vi "temp22100.vi"() -> ()   [LabVIEW 2010]
panel:
  out "Waveform Chart":dbl(graph)
  in  "Boolean":bool
  in  "stop":bool
  in  "Delay Time (s)":dbl=1.0
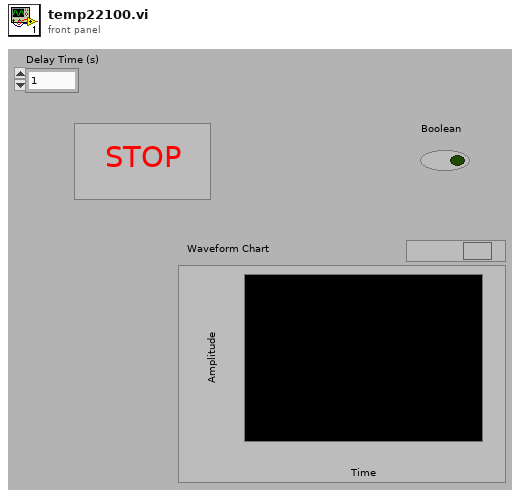
[diagram p1: front panel]
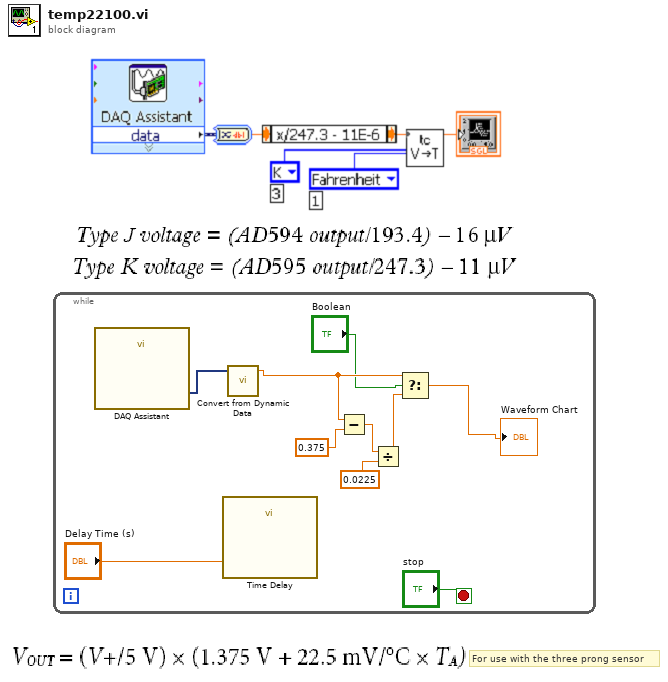
[diagram p0: block diagram]
diagram:
  # "For use with the three prong sensor"
  n1 = while {
    stop <- "stop" stop-if-true
    n2 = call "DAQ Assistant"() -> ("data"=w8:dynamicdata)  [unwired: 17 in, 2 out]
    n3 = call "Time Delay"("Delay Time (s)"="Delay Time (s)") -> ()  [unwired: 10 in, 1 out]
    n4 = call "Convert from Dynamic Data"("Dynamic Data Type"=w8) -> ("Scalar"=w3:dbl)  [unwired: 3 in]
    n5 = Subtract(x=w3, y=0.375) -> (x-y=w6:dbl)
    n6 = Divide(x=w6, y=0.0225) -> (x/y=w4:dbl)
    n7 = Select(t=w3, s="Boolean", f=w4) -> (s? t:f=→"Waveform Chart":dbl)
  }
